vi "Enable Disable Cancel Camera Selection Button.vi"(8 "error in (no error)":errorcluster, 10 "Enable?":bool, 11 "UI in":refnum<class "UI.lvclass">) -> (0 "error out":errorcluster)   [LabVIEW 2020, in "AR Example.lvlib" / "UI.lvclass"]
uses:
  UI.lvclass
  UI.lvclass/UI.ctl
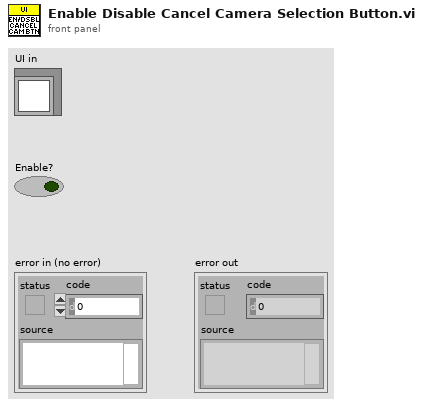
[diagram p1: front panel]
types:
  T1 = enum8{"Enabled", "Disabled", "Disabled and Grayed Out"}
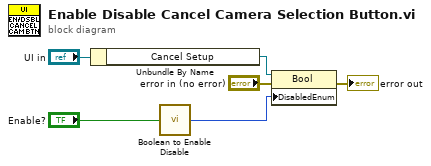
[diagram p0: block diagram]
diagram:
  n1 = Unbundle By Name("UI in") -> ("Cancel Setup"=w5:refnum<vi>)
  n2 = call "Boolean to Enable Disable.vi"("Enable?"="Enable?") -> ("Enable/Disable"=w1:T1)
  n3 = property class="Bool"(reference=w5, error in="error in (no error)", "DisabledEnum"=w1) -> (error out=→"error out":errorcluster)  [unwired: 1 out]
